vi "pack and unpack DRAM data-host.vi"() -> ()   [LabVIEW 2015]
uses:
  <vilib>/rvi/interface/RandomDataEmulation/nirviRandomDataOpen.vi
  <vilib>/rvi/interface/common/niFpgaCacheSessionInfoDynamic.vi
  <vilib>/FPGAPlugInAG/Dynamic/niLvFpga_Reset_Dynamic.vi
  <vilib>/FPGAPlugInAG/Dynamic/niLvFpga_Run_Dynamic.vi
  <vilib>/Utility/error.llb/Error Cluster From Error Code.vi
  <vilib>/rvi/errors/niLvFpgaAdjustHostInterfaceError.vi
  <vilib>/FPGAPlugInAG/Dynamic/niLvFpga_Close_Dynamic.vi
  <vilib>/rvi/interface/nirviOpenFPGA/nirviOpenFPGA.xnode
  Code/LabVIEWcodes/New Codes with SubVIs/Users/OenScan FPGA progrom using Packed data type/Other Test Codes/Pack and unpack DRAM data.vi
  <vilib>/rvi/interface/nirviMethod/nirviMethod.xnode
  <vilib>/rvi/interface/nirviReadWriteControl/nirviReadWriteControl.xnode
  <vilib>/rvi/interface/nirviCloseFPGA/nirviCloseFPGA.xnode
  <vilib>/rvi/errors/niLvFpgaMergeErrorWithErrorCode.vi
  <vilib>/FPGAPlugInAG/Dynamic/niLvFpga_ReadFifo_Dynamic.vi
  NiFpgaLv.dll
  <vilib>/rvi/interface/Simulation/niFpgaSimulationCallBeginRW.vi
  <vilib>/FPGAPlugInAG/Dynamic/niLvFpga_WriteFifo_Dynamic.vi
  <vilib>/FPGAPlugInAG/Dynamic/niLvFpga_StopFifo_Dynamic.vi
panel:
  out "Read DRAM address":u32
  in  "Byte Enables":i64
  out "Array":u32[](array[numeric])
  out "Empty Elements Remaining":u32
  in  "Write DRAM enable?":bool
  out "read DRAM done?":bool
  out "Write DRAM done?":bool
  out "Data readed":u32
  out "Data":u32[](array[numeric])
  in  "Total elements to write":i32
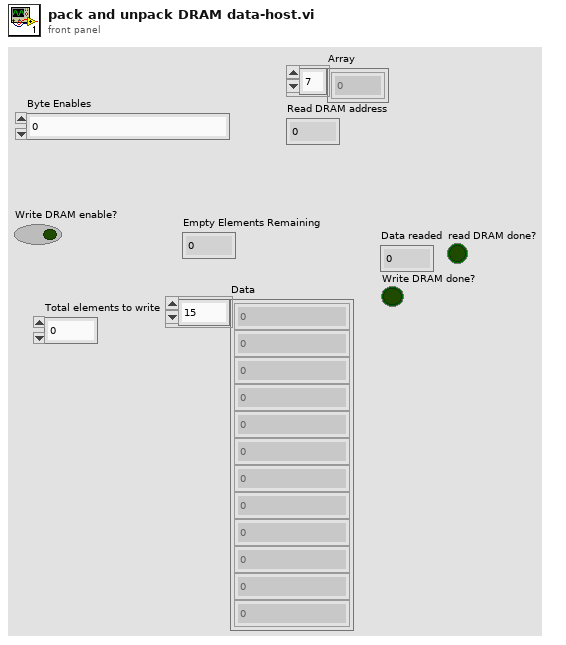
[diagram p1: front panel]
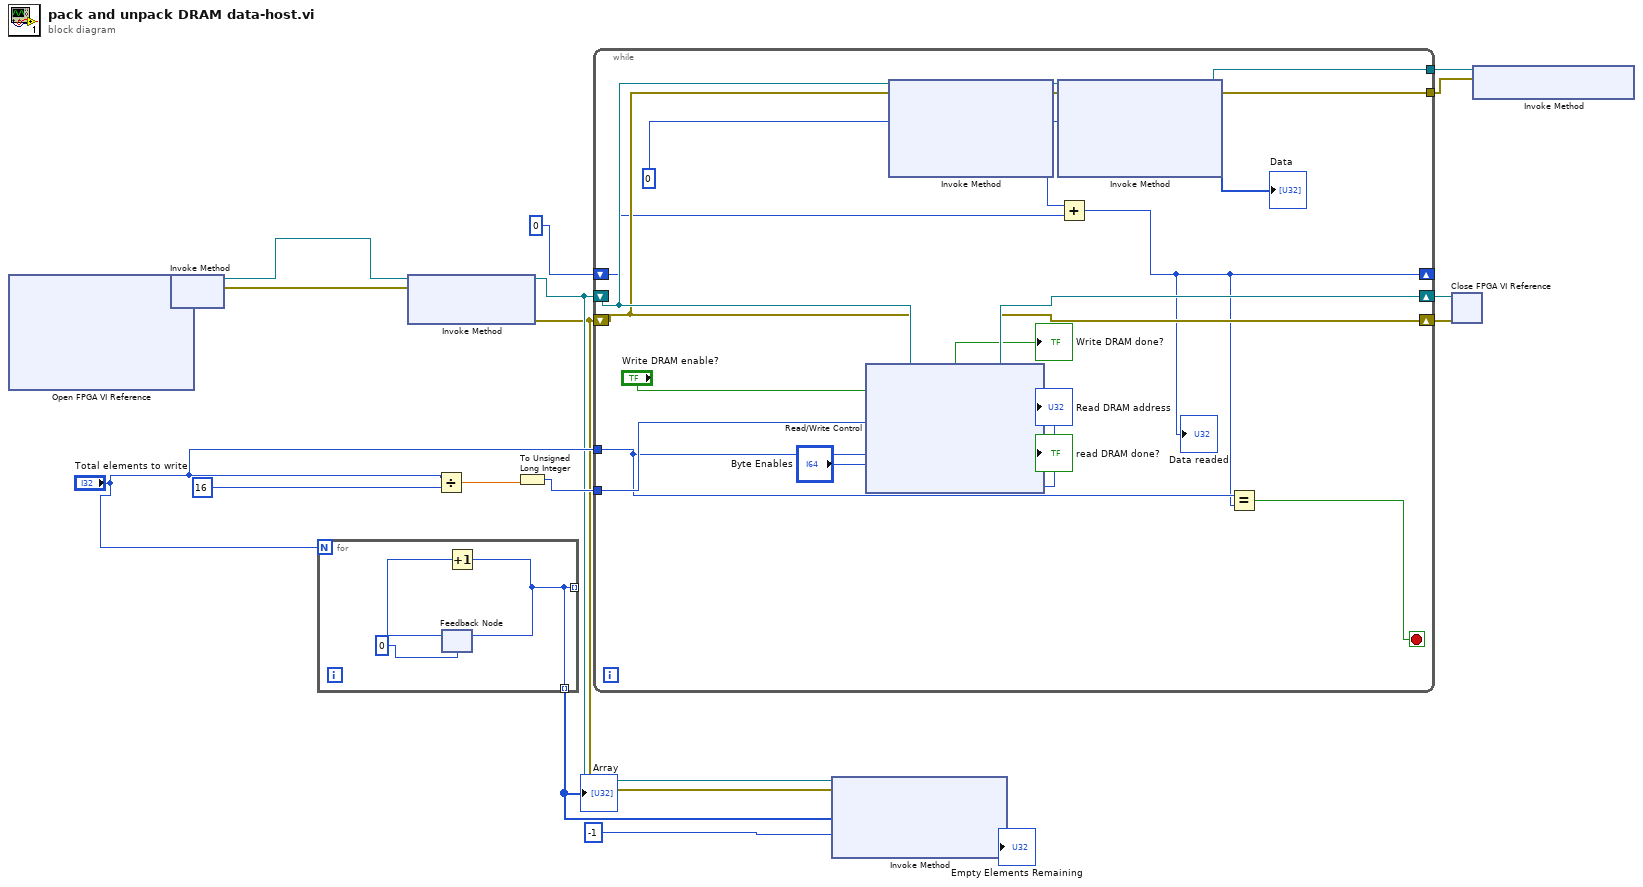
[diagram p0: block diagram]
diagram:
  n1 = xnode "Open FPGA VI Reference"() -> ("FPGA VI引用输出"=w18:refnum<k20>, "错误输出"=w17:errorcluster)  [unwired: 2 in]
  n2 = xnode "Invoke Method"("FPGA VI引用输入"=w18, "错误输入"=w17) -> ("FPGA VI引用输出"=w9:refnum<k20>, "错误输出"=w8:errorcluster)
  n3 = for {
    N: "Total elements to write" -> [_]
    tunnel: [w19] -> _ mode=indexing
    tunnel: [w19] -> w3 mode=indexing
    n4 = feedback #1(u32 0) -> (w21:u32)
    n5 = Increment(x=w21) -> (x+1=w19:u32)
    n6 = feedback-in #1(w19) -> ()
  }
  "Array" <- w3
  n7 = xnode "Invoke Method"("FPGA VI引用输入"=w9, "错误输入"=w8) -> ("FPGA VI引用输出"=w5:refnum<k20>, "错误输出"=w4:errorcluster)  [unwired: 1 in]
  n8 = Divide(x="Total elements to write", y=16) -> (x/y=w13:dbl)
  n9 = To Unsigned Long Integer(number=w13) -> (unsigned 32bit integer=w10:u32)
  n10 = while {
    tunnel: "Total elements to write" -> [w31]
    shift-right: [w42] -> w16
    shift-left: w5 -> [w39]
    shift-right: [w41] -> w15
    shift-left: w4 -> [w38]
    tunnel: w10 -> [w33]
    shift-right: [w26] -> _
    shift-left: u32 0 -> [w27]
    tunnel: [w25] -> w2
    tunnel: [w24] -> w1
    stop <- w30 stop-if-true
    n11 = xnode "Read/Write Control"("FPGA VI引用输入"=w39, "错误输入"=w38, "Write DRAM enable?"="Write DRAM enable?", "Total packed data to write?"=w33, "Total elements to write"=w31, "Byte Enables"="Byte Enables") -> ("FPGA VI引用输出"=w42:refnum<k20>, "错误输出"=w41:errorcluster, "Write DRAM done?"=→"Write DRAM done?":bool, "read DRAM done?"=→"read DRAM done?":bool, "Read DRAM address"=→"Read DRAM address":u32)
    n12 = xnode "Invoke Method"("FPGA VI引用输入"=w39, "错误输入"=w38, "Number of Elements"=u32 0) -> ("FPGA VI引用输出"=w36:refnum<k20>, "错误输出"=w35:errorcluster, "Elements Remaining"=w32:u32)  [unwired: 1 in, 1 out]
    n13 = xnode "Invoke Method"("FPGA VI引用输入"=w36, "错误输入"=w35, "Number of Elements"=w32) -> ("FPGA VI引用输出"=w25:refnum<k20>, "错误输出"=w24:errorcluster, "Data"=→"Data":u32[])  [unwired: 1 in, 1 out]
    n14 = Add(x=w32, y=w27) -> (x+y=w26:u32)
    "Data readed" <- w26
    n15 = Equal?(x=w31, y=w26) -> (x = y?=w30:bool)
  }
  n16 = xnode "Invoke Method"("FPGA VI引用输入"=w5, "错误输入"=w4, "Data"=w3, "Timeout (ms)"=-1) -> ("Empty Elements Remaining"=→"Empty Elements Remaining":u32)  [unwired: 2 out]
  n17 = xnode "Close FPGA VI Reference"("FPGA VI Reference In"=w16, "error in"=w15) -> ()  [unwired: 1 out]
  n18 = xnode "Invoke Method"("FPGA VI引用输入"=w2, "错误输入"=w1) -> ()  [unwired: 2 out]
